vi "Display Type PN.vi"(8 "error in":errorcluster, 10 "s? t:f":u32, 11 "reference":refnum<vi>) -> (0 "error out":errorcluster, 3 "reference out":refnum<vi>)   [LabVIEW 2022 SP3]
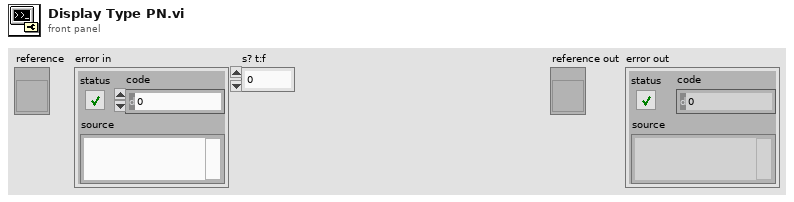
[diagram p1: front panel]
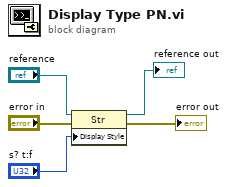
[diagram p0: block diagram]
diagram:
  n1 = property class="Str"(reference="reference", error in="error in", "Display Style"="s? t:f") -> (reference out=→"reference out":refnum<vi>, error out=→"error out":errorcluster)
